vi "Write_Data_INI.vi"(0 "Application_Directory":path, 2 "Section":string, 5 "File_Name":path, 7 "Data":string, 11 "Error_In":errorcluster, 13 "Key":string) -> (4 "File_Path_Out":path, 15 "Error_Out":errorcluster)   [LabVIEW 2021]
doc: "This VI write data to ini file"
uses:
  <vilib>/Utility/config.llb/NI_LVConfig.lvlib
  <vilib>/Utility/config.llb/Write Key (String).vi
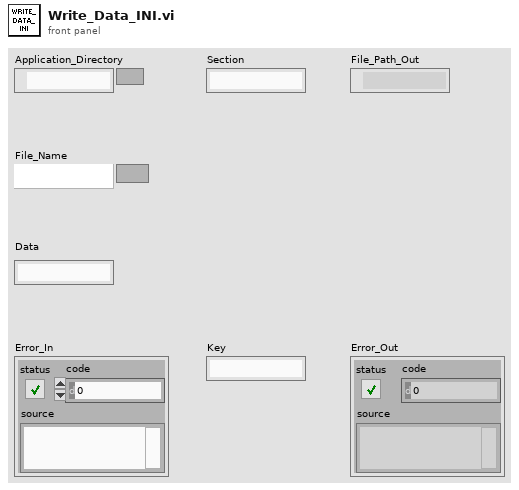
[diagram p1: front panel]
types:
  T1 = typedef "NI_LVConfig.lvlib/Config Data RefNum.ctl" = refnum<k1>
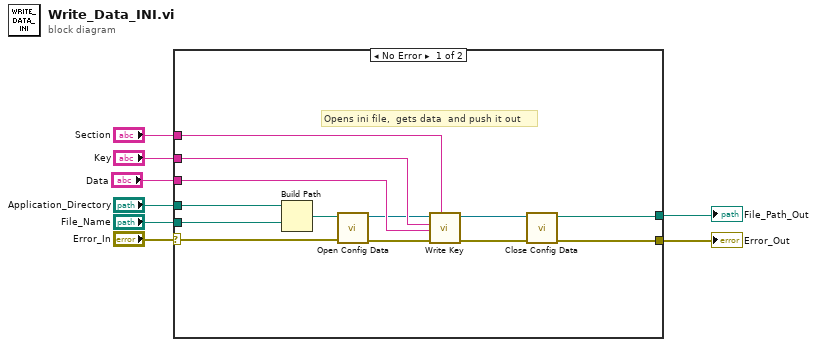
[diagram p0: block diagram]
diagram:
  n1 = case shown="No Error" "Error_In" {
    selector: "Error_In" -> [w16 w23]
    tunnel: "Application_Directory" -> [w20 w22]
    tunnel: "Key" -> [w18 _]
    tunnel: "Section" -> [w17 _]
    tunnel: [w15 w23] -> w4
    tunnel: [w14 w22] -> w3
    tunnel: "File_Name" -> [w13 _]
    tunnel: "Data" -> [w10 _]
    frame No Error {
      # "Opens ini file,  gets data  and push it out"
      n2 = Build Path(base path=w20, name or relative path=w13) -> (appended path=w19:path)
      n3 = call <vilib>:"Open Config Data.vi"("error in (no error)"=w16, "configuration file path"=w19) -> ("error out"=w11:errorcluster, "refnum"=w9:T1)  [unwired: 7 in, 1 out]
      n4 = call-poly <vilib>:"Write Key.vi"("section"=w17, "error in (no error)"=w11, "value"=w10, "key"=w18, "refnum"=w9) -> ("error out"=w21:errorcluster, "refnum out"=w12:T1)  [unwired: 4 in, 1 out]
      n5 = call <vilib>:"Close Config Data.vi"("error in (no error)"=w21, "refnum"=w12) -> ("error out"=w15:errorcluster, "file path"=w14:path)  [unwired: 8 in]
    }
    frame Error {
    }
  }
  "Error_Out" <- w4
  "File_Path_Out" <- w3
